vi "Write currentTimes.vi"(8 "error in (no error)":errorcluster, 10 "CurrentTimes.lvclass":refnum<class "CurrentTimes.lvclass">, 11 "TCSPublicStatus in":refnum<class "TCSTcsStatus.lvclass">) -> (0 "error out":errorcluster, 3 "TCSPublicStatus out":refnum<class "TCSTcsStatus.lvclass">)   [LabVIEW 2022 SP3, in "TCSDataDefinitions.lvlib" / "TCSPublicStatus.lvlib" / "TCSTcsStatus.lvclass"]
uses:
  TCSTcsStatus.lvclass
  CurrentTimes/CurrentTimes/CurrentTimes.lvclass
  TCSTcsStatus.lvclass/TCSTcsStatus.ctl
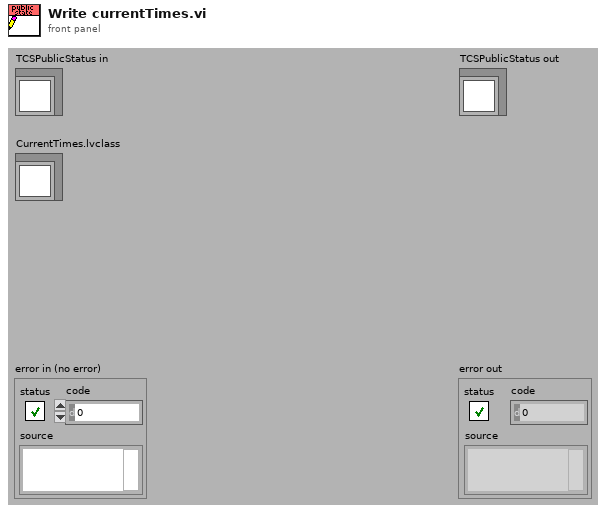
[diagram p1: front panel]
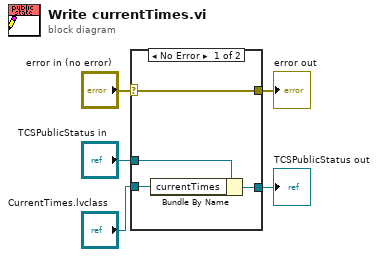
[diagram p0: block diagram]
diagram:
  n1 = case shown="No Error" "error in (no error)" {
    selector: "error in (no error)" -> [w9 w10]
    tunnel: [w9 w10] -> w4
    tunnel: [w7 w11] -> w2
    tunnel: "TCSPublicStatus in" -> [w8 w11]
    tunnel: "CurrentTimes.lvclass" -> [w6 _]
    frame No Error {
      n2 = Bundle By Name(cluster=w8, "currentTimes"=w6) -> (w7:refnum<class "TCSTcsStatus.lvclass">)
    }
    frame Error {
    }
  }
  "error out" <- w4
  "TCSPublicStatus out" <- w2
